vi "Write Unit ID.vi"(8 "error in (no error)":errorcluster, 10 "unit ID":u8, 11 "Modbus instance in":refnum<class "Modbus API.lvclass">) -> (0 "error out":errorcluster, 3 "Modbus instance out":refnum<class "Modbus API.lvclass">)   [LabVIEW 2021]
doc: "Sets the unit ID of the device."
uses:
  Modbus API.lvclass/Modbus API.ctl
  Transmission Data Unit/Transmission Data Unit.lvclass
  Network Protocol/Network Protocol.lvclass
  Modbus API.lvclass
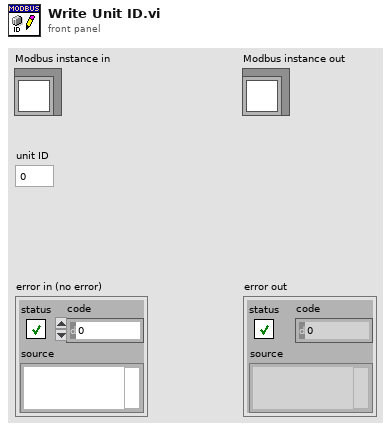
[diagram p1: front panel]
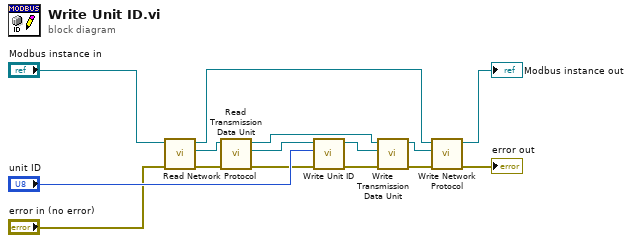
[diagram p0: block diagram]
diagram:
  n1 = call "Read Network Protocol.vi"("error in (no error)"="error in (no error)", "Modbus API in"="Modbus instance in") -> ("error out"=w11:errorcluster, "Network Protocol"=w8:refnum<class "Network Protocol.lvclass">, "Modbus API out"=w2:refnum<class "Modbus API.lvclass">)  [unwired: 7 in]
  n2 = call "Read Transmission Data Unit.vi"("error in (no error)"=w11, "Network Protocol in"=w8) -> ("error out"=w9:errorcluster, "Transmission Data Unit"=w14:refnum<class "Transmission Data Unit.lvclass">, "Network Protocol out"=w6:refnum<class "Network Protocol.lvclass">)  [unwired: 7 in]
  n3 = call "Write Unit ID.vi"("error in"=w9, "unit ID"="unit ID", "transmission data unit in"=w14) -> ("error out"=w4:errorcluster, "transmission data unit out"=w13:refnum<class "Transmission Data Unit.lvclass">)  [unwired: 7 in]
  n4 = call "Write Transmission Data Unit.vi"("error in (no error)"=w4, "Transmission Data Unit"=w13, "Network Protocol in"=w6) -> ("error out"=w5:errorcluster, "Network Protocol out"=w7:refnum<class "Network Protocol.lvclass">)  [unwired: 7 in]
  n5 = call "Write Network Protocol.vi"("error in (no error)"=w5, "Network Protocol"=w7, "Modbus API in"=w2) -> ("error out"=→"error out":errorcluster, "Modbus API out"=→"Modbus instance out":refnum<class "Modbus API.lvclass">)  [unwired: 7 in]
